vi "WeatherMapAPI_Read Config File Parameters.vi"(8 "error in":errorcluster) -> (0 "error out":errorcluster, 3 "API Key out":string)   [LabVIEW 2021]
uses:
  <vilib>/Utility/config.llb/Read Key (String).vi
  <vilib>/Utility/config.llb/NI_LVConfig.lvlib
panel:
  out "Cfg file path":path
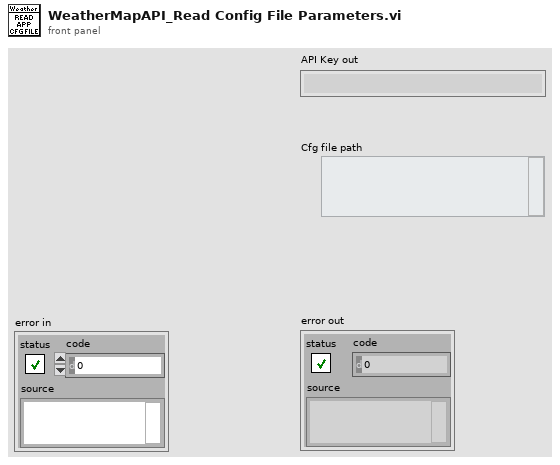
[diagram p1: front panel]
types:
  T1 = typedef "NI_LVConfig.lvlib/Config Data RefNum.ctl" = refnum<k1>
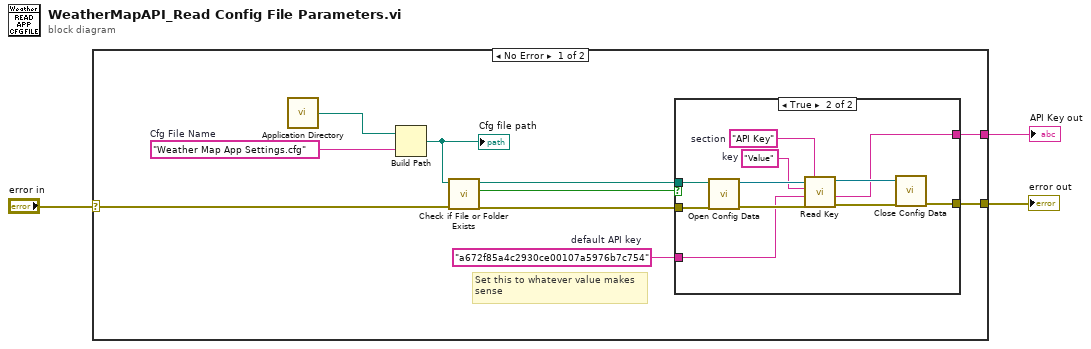
[diagram p0: block diagram]
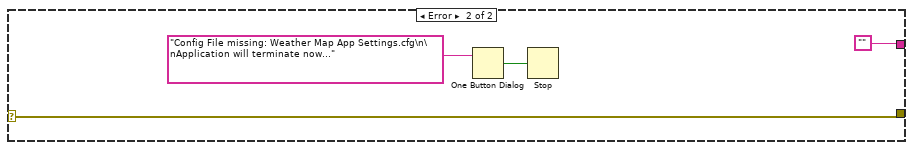
[diagram p3: hidden frame]
diagram:
  n1 = case shown="No Error" "error in" {
    selector: "error in" -> [w4 w30]
    tunnel: [w12 ""] -> w3
    tunnel: [w11 w30] -> w2
    frame No Error {
      w7 = "Weather Map App Settings.cfg"  # Cfg File Name
      w13 = "a672f85a4c2930ce00107a5976b7c754"  # default API key
      # "Set this to whatever value makes\nsense"
      n2 = call <vilib>:"Application Directory.vi"() -> ("Application Directory"=w6:path)
      n3 = Build Path(base path=w6, name or relative path=w7) -> (appended path=w5:path)
      "Cfg file path" <- w5
      n4 = call <vilib>:"Check if File or Folder Exists.vi"("error in (no error)"=w4, "path"=w5) -> ("error out"=w10:errorcluster, "file or folder exists?"=w8:bool, "dup path"=w9:path)  [unwired: 7 in]
      n5 = case shown="True" w8 {
        tunnel: w13 -> [w14 w22]
        tunnel: [w14 w19] -> w12
        tunnel: [w15 w18] -> w11
        tunnel: w10 -> [w15 w17]
        tunnel: w9 -> [_ w16]
        frame False {
        }
        frame True {
          w20 = "Value"  # key
          w21 = "API Key"  # section
          n6 = call <vilib>:"Open Config Data.vi"("error in (no error)"=w17, "configuration file path"=w16) -> ("error out"=w26:errorcluster, "refnum"=w25:T1)  [unwired: 7 in, 1 out]
          n7 = call-poly <vilib>:"Read Key.vi"("section"=w21, "error in (no error)"=w26, "default value"=w22, "key"=w20, "refnum"=w25) -> ("error out"=w24:errorcluster, "value"=w19:string, "refnum out"=w23:T1)  [unwired: 3 in, 1 out]
          n8 = call <vilib>:"Close Config Data.vi"("error in (no error)"=w24, "refnum"=w23) -> ("error out"=w18:errorcluster)  [unwired: 8 in, 1 out]
        }
      }
    }
    frame Error {
      n9 = One Button Dialog(message="Config File missing: Weather Map App Settings.cfg\n\nApplication will terminate now...") -> (true=w27:bool)  [unwired: 1 in]
      n10 = Stop(stop? (T)=w27) -> ()
    }
  }
  "API Key out" <- w3
  "error out" <- w2
